vi "WPI_DashboardPadding for Joystick Buttons.vi"(11 "Array":u8[](array[numeric])) -> (3 "Boolean array":bool[](array[boolean]))   [LabVIEW 2025]
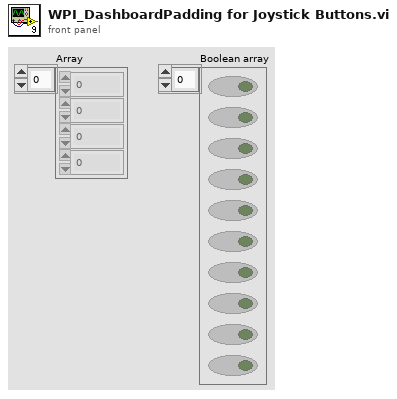
[diagram p1: front panel]
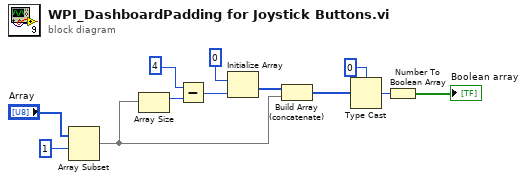
[diagram p0: block diagram]
diagram:
  n1 = Array Subset(array="Array", index=1) -> (w1:u8[])  [unwired: 1 in]
  n2 = Array Size(array=w1) -> (size(s)=w7:i32)
  n3 = Subtract(x=4, y=w7) -> (x-y=w5:i32)
  n4 = Initialize Array(u8 0, w5) -> (w3:u8[])
  n5 = Build Array (concatenate)(w3, w1) -> (w2:u8[])
  n6 = Type Cast(type=0, x=w2) -> (*(type *) &x=w10:i32)
  n7 = Number To Boolean Array(number=w10) -> (Boolean array=→"Boolean array":bool[])
